vi "ClientLabView_Victor.vi"() -> ()   [LabVIEW 2014]
uses:
  Control 1.ctl
panel:
  in  "Nombre de mostres mitjana":dbl=1.0 min=1.0 max=9.0 step=1.0
  in  "Temps de mostratge":dbl=1.0 min=1.0 max=20.0 step=1.0
  in  "Missatge a enviar":T1="No enviar res"
  in  "Botó per enviar":bool
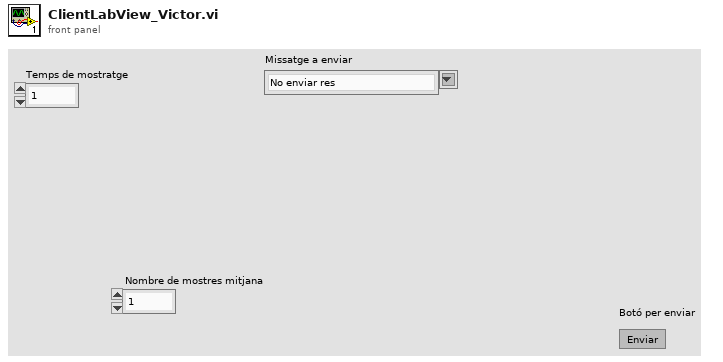
[diagram p1: front panel]
types:
  T1 = typedef "Control 1.ctl" = string
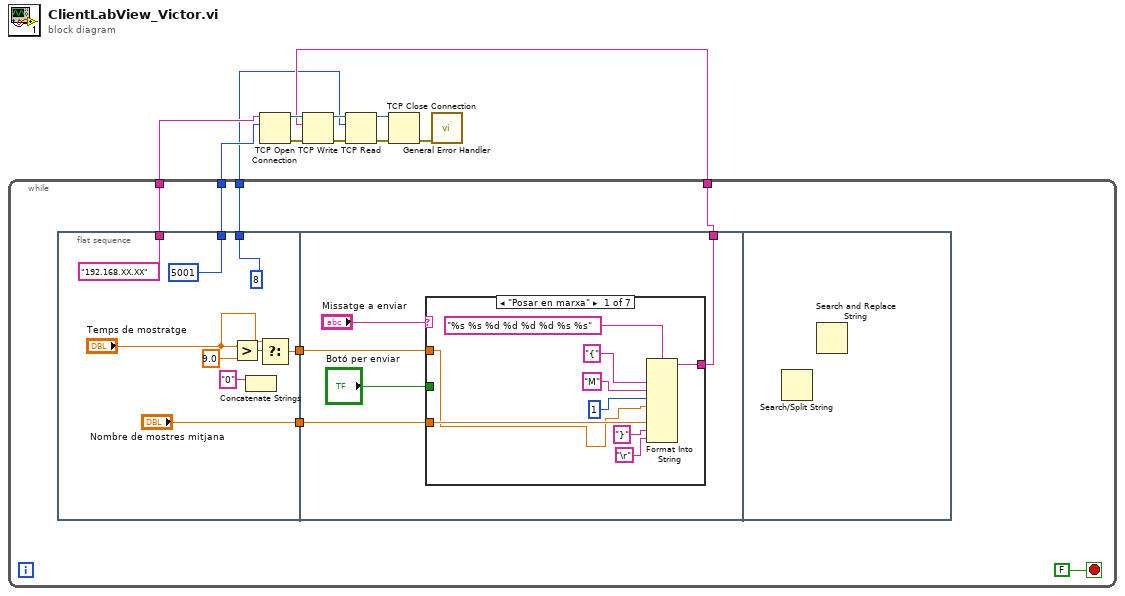
[diagram p0: block diagram]
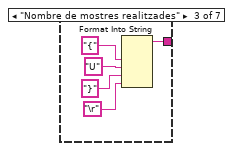
[diagram p3: hidden frame]
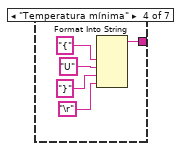
[diagram p4: hidden frame]
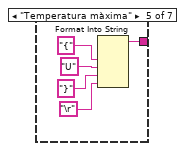
[diagram p5: hidden frame]
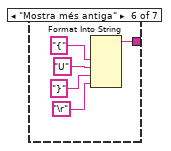
[diagram p6: hidden frame]
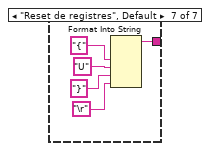
[diagram p7: hidden frame]
diagram:
  n1 = while {
    tunnel: [w17] -> w4
    tunnel: [w14] -> w3
    tunnel: [w13] -> w2
    tunnel: [w12] -> w1
    stop <- FALSE stop-if-true
    n2 = flat-sequence {
      tunnel: ["Nombre de mostres mitjana"] -> w16
      tunnel: [w26] -> w15
      tunnel: ["192.168.XX.XX"] -> w14
      tunnel: [5001] -> w13
      tunnel: [8] -> w12
      tunnel: [w31] -> w17
      tunnel: w16 -> [w30]
      tunnel: w15 -> [w28]
      frame #0 {
        n3 = Greater?(x="Temps de mostratge", y=9.0) -> (0:w23:bool)
        n4 = Concatenate Strings("0" ("string")) -> ()  [unwired: 1 in, 1 out]
        n5 = Select(t="Temps de mostratge", s=w23) -> (s? t:f=w26:dbl)  [unwired: 1 in]
      }
      frame #1 {
        n6 = case shown="\"Posar en marxa\"" "Missatge a enviar" {
          tunnel: [w39 _ w42 w47 w52 w57 w62] -> w31
          tunnel: w30 -> [w34 _ _ _ _ _ _]
          tunnel: "Botó per enviar" -> [_ _ _ _ _ _ _]
          tunnel: w28 -> [w33 _ _ _ _ _ _]
          frame "Posar en marxa" {
            n7 = Format Into String(format string="%s %s %d %d %d %d %s %s", "{", "M", 1 ("input 3"), w33, w34, "}", "\r") -> (resulting string=w39:string)  [unwired: 3 in, 1 out]
          }
          frame "Atura" {
          }
          frame "Nombre de mostres realitzades" {
            n8 = Format Into String("{", "U", "}", "\r") -> (resulting string=w42:string)  [unwired: 3 in, 1 out]
          }
          frame "Temperatura mínima" {
            n9 = Format Into String("{", "U", "}", "\r") -> (resulting string=w47:string)  [unwired: 3 in, 1 out]
          }
          frame "Temperatura màxima" {
            n10 = Format Into String("{", "U", "}", "\r") -> (resulting string=w52:string)  [unwired: 3 in, 1 out]
          }
          frame "Mostra més antiga" {
            n11 = Format Into String("{", "U", "}", "\r") -> (resulting string=w57:string)  [unwired: 3 in, 1 out]
          }
          frame "Reset de registres", Default {
            n12 = Format Into String("{", "U", "}", "\r") -> (resulting string=w62:string)  [unwired: 3 in, 1 out]
          }
        }
      }
      frame #2 {
        n13 = Search/Split String() -> ()  [unwired: 3 in, 3 out]
        n14 = Search and Replace String() -> ()  [unwired: 8 in, 4 out]
      }
    }
  }
  n15 = TCP Open Connection(address=w3, remote port or service name=w2) -> (connection ID=w11:refnum<k5>, error out=w8:errorcluster)  [unwired: 3 in]
  n16 = TCP Write(connection ID=w11, data in=w4, error in (no error)=w8) -> (connection ID out=w10:refnum<k5>, error out=w7:errorcluster)  [unwired: 1 in, 1 out]
  n17 = TCP Read(connection ID=w10, bytes to read=w1, error in (no error)=w7) -> (connection ID out=w9:refnum<k5>, error out=w6:errorcluster)  [unwired: 2 in, 1 out]
  n18 = TCP Close Connection(connection ID=w9, error in (no error)=w6) -> (error out=w5:errorcluster)  [unwired: 1 in, 1 out]
  n19 = call <vilib>:"General Error Handler.vi"("error in (no error)"=w5) -> ()  [unwired: 10 in, 5 out]
